vi "Paskevits_Vladislav_gbl.vi"() -> ()   [LabVIEW 2018]
doc: "This GlobalVariable should stop the main programm"
panel:
  in  "stop":bool
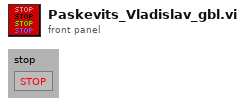
[diagram p1: front panel]
diagram:
